vi "XML_EEG_anythingToHexString.vi"   [LabVIEW 2016, in "XML_EEG_File_Parser.lvlib"]
uses:
  XML_EEG_File_Parser.lvlib
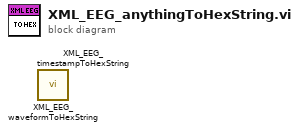
[diagram p0: block diagram]
diagram:
  n1 = call "XML_EEG_waveformToHexString.vi"() -> ()  [unwired: 10 in, 2 out]
  n2 = call "XML_EEG_timestampToHexString.vi"() -> ()  [unwired: 10 in, 2 out]
